vi "upload_file.vi"(8 "error in (no error)":errorcluster, 9 "file":string, 10 "path":string, 11 "filepath":path) -> (0 "error out":errorcluster, 3 "filepath":string)   [LabVIEW 2015, in "lv-dropbox.lvlib" / "v2.lvlib"]
uses:
  v2.lvlib
  private/_controls/content_type.ctl
  <vilib>/httpClient/POSTBuffer.vi
  <vilib>/httpClient/LabVIEWHTTPClient.lvlib
  lv-dropbox.lvlib
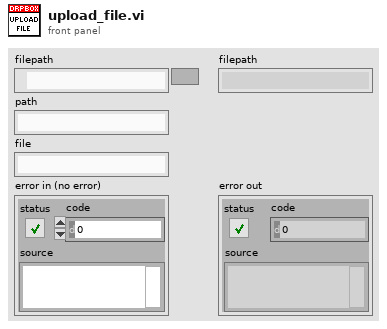
[diagram p1: front panel]
types:
  T1 = typedef "lv-dropbox.lvlib/content_type.ctl" = enum16{"<content_type>", "application/json", "application/octet-stream", "application/x-www-form-urlencoded"}
  T2 = cluster{"name":string, "path_lower":string, "id":string, "client_modified":string, "server_modified":string, "rev":string, "size":u64}
  T3 = typedef "LabVIEWHTTPClient.lvlib/ClientHandle.ctl" = refnum<k1>
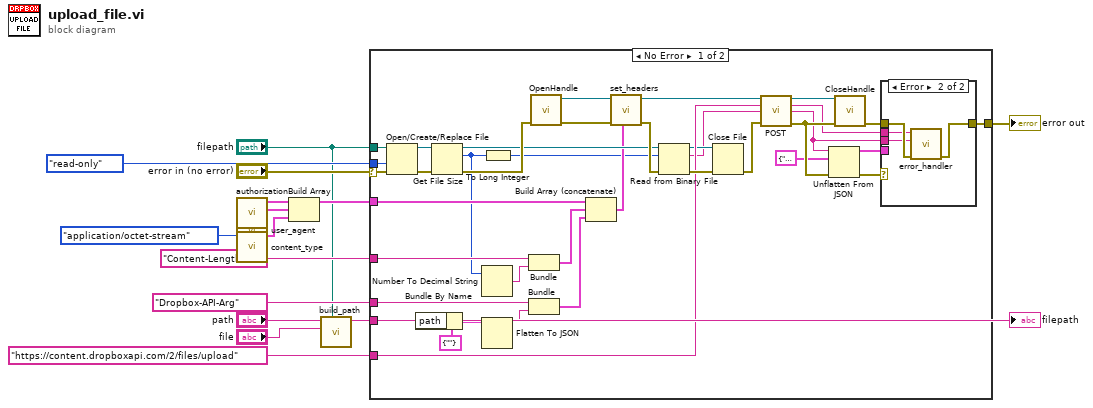
[diagram p0: block diagram]
diagram:
  n1 = call "authorization.vi"() -> ("header"=w12:cluster{"header":string, "value":string})  [unwired: 11 in]
  n2 = call "user_agent.vi"() -> ("header"=w11:cluster{"header":string, "value":string})  [unwired: 11 in]
  n3 = call "content_type.vi"("content_type"=content_type."application/octet-stream") -> ("header"=w13:cluster{"header":string, "value":string})  [unwired: 10 in]
  n4 = Build Array(w12, w11, w13) -> (w7:cluster{"header":string, "value":string}[])
  n5 = call "build_path.vi"("filepath"="filepath", "path"="file", "base_path"="path") -> ("path"=w2:string)  [unwired: 8 in]
  "filepath" <- w2
  n6 = case shown="No Error" "error in (no error)" {
    selector: "error in (no error)" -> [w49 w59]
    tunnel: enum16{"read/write", "read-only", "write-only"}."read-only" ("access (0:read/write)") -> [w48 _]
    tunnel: "Dropbox-API-Arg" ("header") -> [w47 _]
    tunnel: "Content-Length" ("header") -> [w46 _]
    tunnel: w7 -> [w45 _]
    tunnel: "https://content.dropboxapi.com/2/files/upload" ("url") -> [w44 _]
    tunnel: [w43 w59] -> w5
    tunnel: "filepath" -> [w17 _]
    tunnel: w2 -> [w16 _]
    frame No Error {
      n7 = Open/Create/Replace File(file path (use dialog)=w17, error in=w49, access (0:read/write)=w48) -> (refnum out=w38:refnum<file>, error out=w41:errorcluster)  [unwired: 3 in, 1 out]
      n8 = Bundle By Name(cluster=cluster{"path":string} {"path"=""}, "path"=w16) -> (w35:cluster{"path":string})
      n9 = Get File Size(file=w38, error in=w41) -> (refnum out=w40:refnum<file>, size (in bytes)=w39:i64, 0:w53:errorcluster)
      n10 = Number To Decimal String(number=w39) -> (decimal integer string=w42:string)  [unwired: 1 in]
      n11 = Flatten To JSON(anything=w35) -> (JSON string=w31:string)  [unwired: 2 in, 1 out]
      n12 = To Long Integer(number=w39) -> (32bit integer=w21:i32)
      n13 = Bundle("header"=w46, w42) -> (w20:cluster{"header":string, string})  [unwired: 1 in]
      n14 = Bundle("header"=w47, "JSON string"=w31) -> (w19:cluster{"header":string, "JSON string":string})  [unwired: 1 in]
      n15 = call <vilib>:"OpenHandle.vi"("error in (no error)"=w53) -> ("client handle out"=w32:T3, "error out"=w18:errorcluster)  [unwired: 13 in]
      n16 = Build Array (concatenate)(w45, w20, w19) -> (w29:cluster{"header":string, "JSON string":string}[])
      n17 = call "set_headers.vi"("header_value []"=w29, "error in (no error)"=w18, "client_handle in"=w32) -> ("error out"=w50:errorcluster, "client_handle out"=w30:T3)  [unwired: 7 in]
      n18 = Read from Binary File(8:w50, 10:w21, 11:w40) -> (0:w52:errorcluster, 2:w27:string, 3:w28:refnum<file>)  [unwired: 3 in, 1 out]
      n19 = Close File(refnum=w28, error in=w52) -> (error out=w51:errorcluster)  [unwired: 1 out]
      n20 = call-poly <vilib>:"POST.vi"("client handle"=w30, "url"=w44, "buffer"=w27, "error in (no error)"=w51) -> ("client handle out"=w34:T3, "headers"=w23:string, "body"=w22:string, "error out"=w37:errorcluster)  [unwired: 8 in]
      n21 = Unflatten From JSON(JSON string=w22, type and defaults=T2 {"name"="", "path_lower"="", "id"="", "client_modified"="", "server_modified"="", "rev"="", "size"=0}, error in (no error)=w37) -> (value=w25:T2, error out=w26:errorcluster)  [unwired: 4 in]
      n22 = call <vilib>:"CloseHandle.vi"("client handle"=w34, "error in (no error)"=w37) -> ("error out"=w24:errorcluster)  [unwired: 13 in]
      n23 = case shown="Error" w26 {
        tunnel: w25 -> [_ _]
        tunnel: w24 -> [w54 w58]
        tunnel: [w54 w57] -> w43
        tunnel: w23 -> [_ w56]
        tunnel: w22 -> [_ w55]
        frame No Error {
        }
        frame Error {
          n24 = call "error_handler.vi"("error in (no error)"=w58, "body"=w55, "headers"=w56) -> ("error out"=w57:errorcluster)  [unwired: 8 in]
        }
      }
    }
    frame Error {
    }
  }
  "error out" <- w5
